vi "Build Message Configuration.vi"(8 "error in (no error)":errorcluster, 11 "Message XML Node":refnum<k20>) -> (0 "error out":errorcluster, 2 "Message  Config":T7={"Time to Next Msg (4 us)"=100, "Command Config"={"Command Type"=enum."Transmit", "Terminal Address"=enum."0", "SubAddress"=enum."Mode Code", "Word Count\\Mode Code"=enum."1", "Command Data"=[]}, "Message Control"={"MC17 Time Sync"=FALSE, "Error Mask"=FALSE, "Service Request Mask"=FALSE, "Busy Mask"=FALSE, "SubSystem Flag Mask"=FALSE, "Terminal Flag Mask"=FALSE, "Reserved Mask"=FALSE, "Retry"=FALSE, "Bus A / !Bus B"=FALSE, "Self-Test Loopback"=FALSE, "Broadcast Mask"=FALSE, "EoM Interrupt"=FALSE, "Mode Code Format"=FALSE, "Broadcast Format"=FALSE, "RT-RT Format"=FALSE}}, 3 "RT-RT Message Config":T1, 4 "RT-RT?":bool, 6 "Async?":bool)   [LabVIEW 2020]
doc: "Builds the various different flavors of Messages that can be defined by the XML. All Message types are handled here, including Asynchronous messages."
uses:
  Frames & Messages/TypeDefs/Message Config.ctl
  Frames & Messages/TypeDefs/Command Config.ctl
  Frames & Messages/TypeDefs/Command Type.ctl
  Frames & Messages/TypeDefs/Command Terminal Address.ctl
  Frames & Messages/TypeDefs/Command SubAddress.ctl
  Frames & Messages/TypeDefs/Command Word Count.ctl
  Frames & Messages/TypeDefs/Message Control.ctl
  Frames & Messages/TypeDefs/RT-RT Message Config.ctl
  BCI-1553 API.lvlib
  <vilib>/xml/NI_XML.lvlib
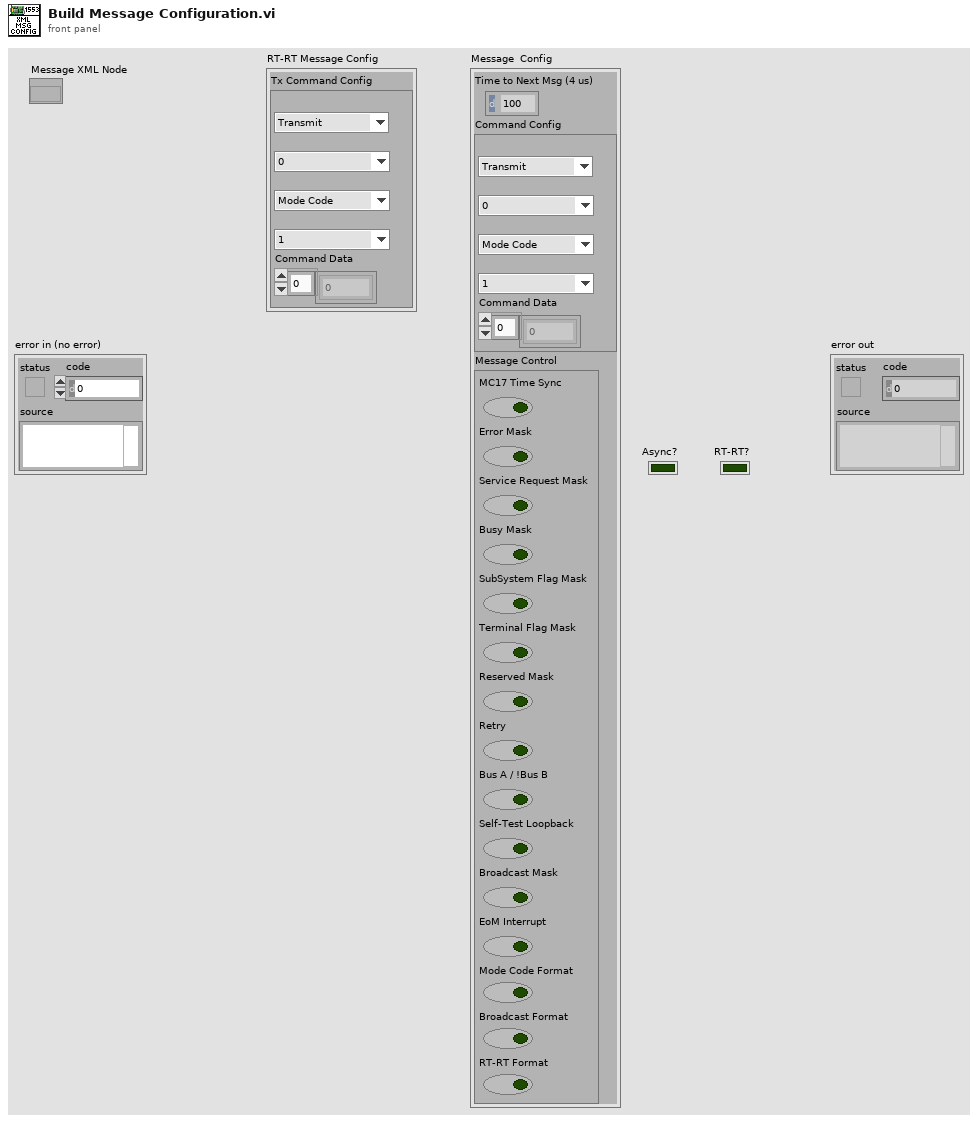
[diagram p1: front panel]
types:
  T1 = typedef "BCI-1553 API.lvlib/RT-RT Message Config.ctl" = cluster{"Tx Command Config":T2}
  T2 = typedef "BCI-1553 API.lvlib/Command Config.ctl" = cluster{"Command Type":T3, "Terminal Address":T4, "SubAddress":T5, "Word Count\\Mode Code":T6, "Command Data":u16[]}
  T3 = typedef "BCI-1553 API.lvlib/Command Type.ctl" = enum16{"Transmit", "Receive"}
  T4 = typedef "BCI-1553 API.lvlib/Command Terminal Address.ctl" = enum16{"0", "1", "2", "3", "4", "5", "6", "7", "8", "9", "10", "11", "12", "13", "14", "15", "16", "17", "18", "19", "20", "21", "22", "23", "24", "25", "26", "27", "28", "29", "30", "Broadcast"}
  T5 = typedef "BCI-1553 API.lvlib/Command SubAddress.ctl" = enum16{"Mode Code", "1", "2", "3", "4", "5", "6", "7", "8", "9", "10", "11", "12", "13", "14", "15", "16", "17", "18", "19", "20", "21", "22", "23", "24", "25", "26", "27", "28", "29", "30"}
  T6 = typedef "BCI-1553 API.lvlib/Command Word Count.ctl" = enum16{"1", "2", "3", "4", "5", "6", "7", "8", "9", "10", "11", "12", "13", "14", "15", "16", "17", "18", "19", "20", "21", "22", "23", "24", "25", "26", "27", "28", "29", "30", "31", "32"}
  T7 = typedef "BCI-1553 API.lvlib/Message Config.ctl" = cluster{"Time to Next Msg (4 us)":u16, "Command Config":T2, "Message Control":T8}
  T8 = typedef "BCI-1553 API.lvlib/Message Control.ctl" = cluster{"MC17 Time Sync":bool, "Error Mask":bool, "Service Request Mask":bool, "Busy Mask":bool, "SubSystem Flag Mask":bool, "Terminal Flag Mask":bool, "Reserved Mask":bool, "Retry":bool, "Bus A / !Bus B":bool, "Self-Test Loopback":bool, "Broadcast Mask":bool, "EoM Interrupt":bool, "Mode Code Format":bool, "Broadcast Format":bool, "RT-RT Format":bool}
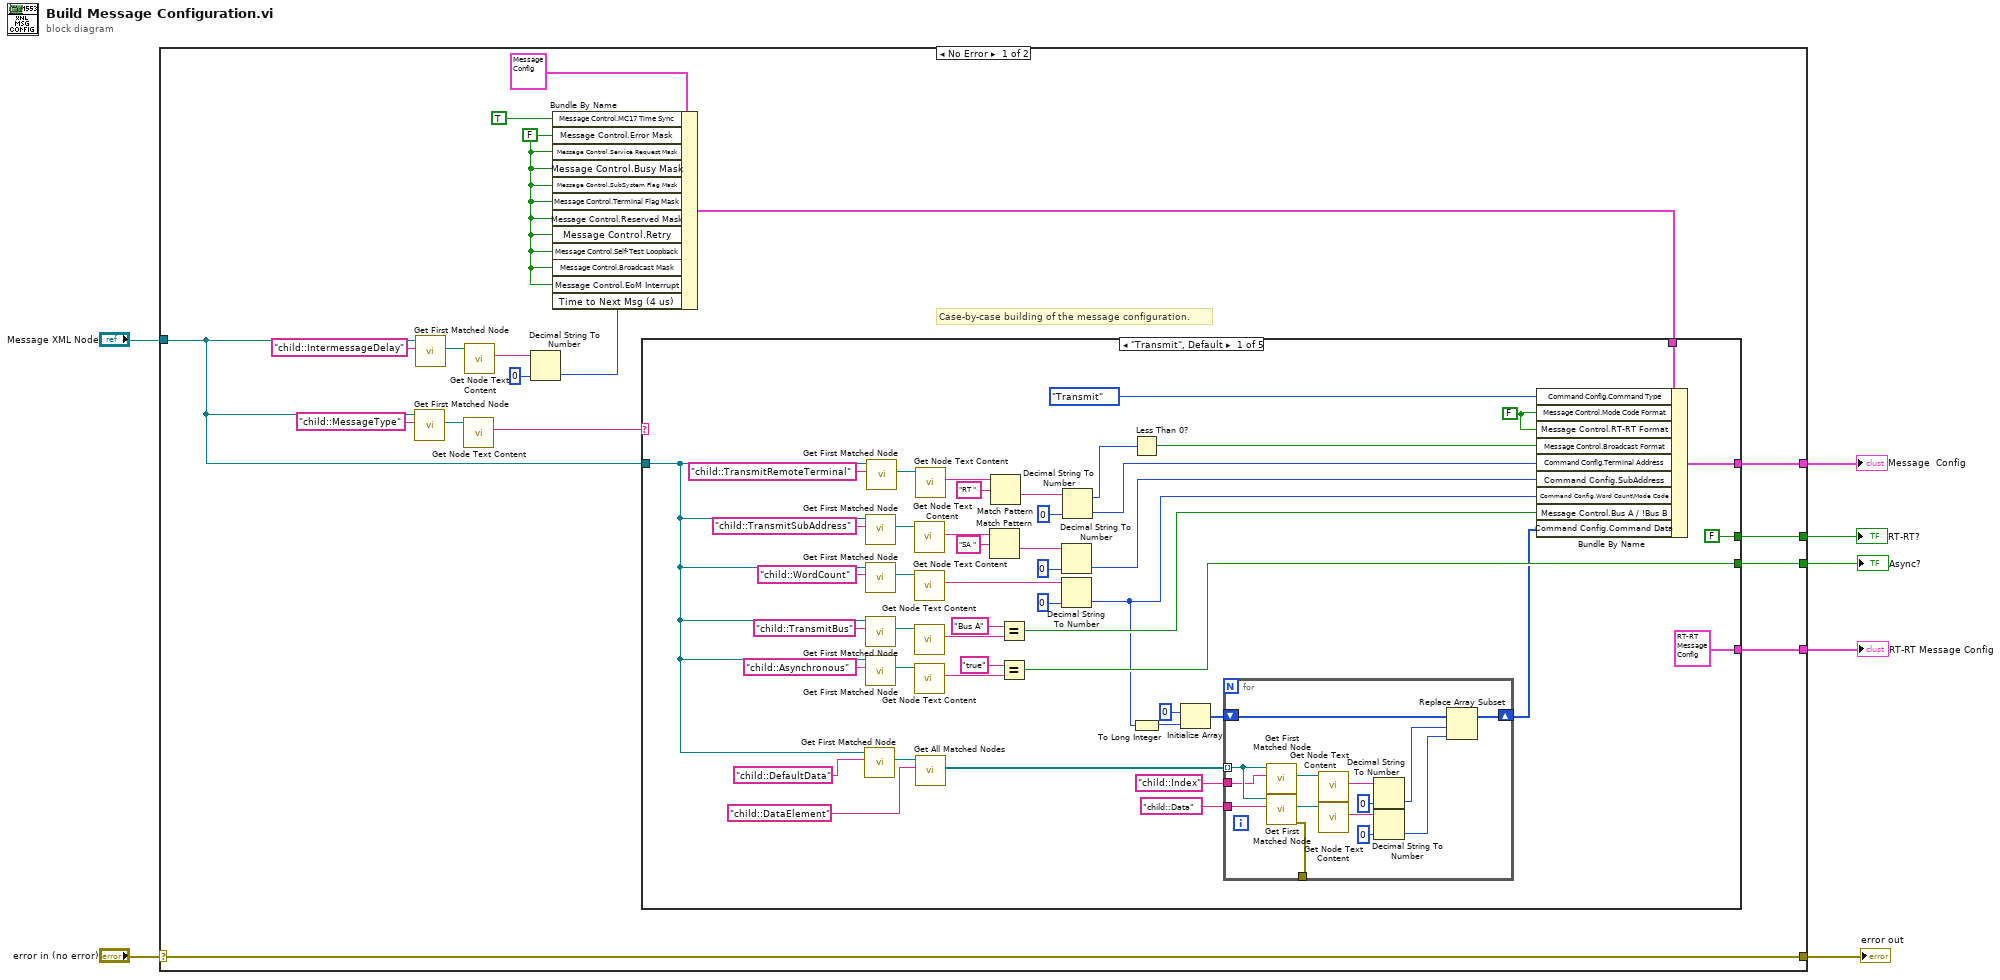
[diagram p0: block diagram]
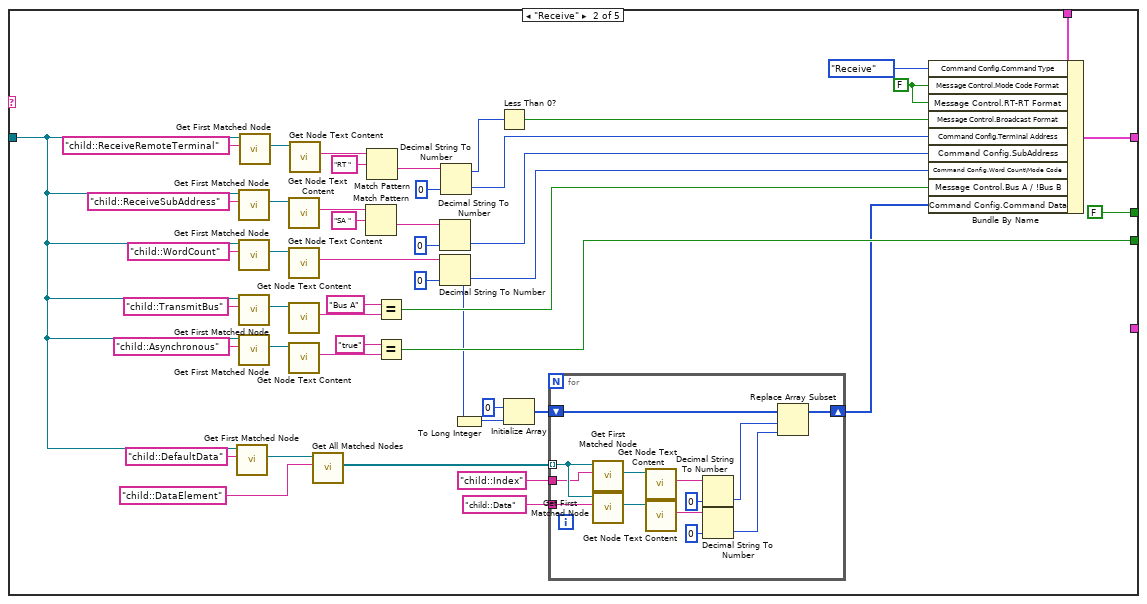
[diagram p2: hidden frame]
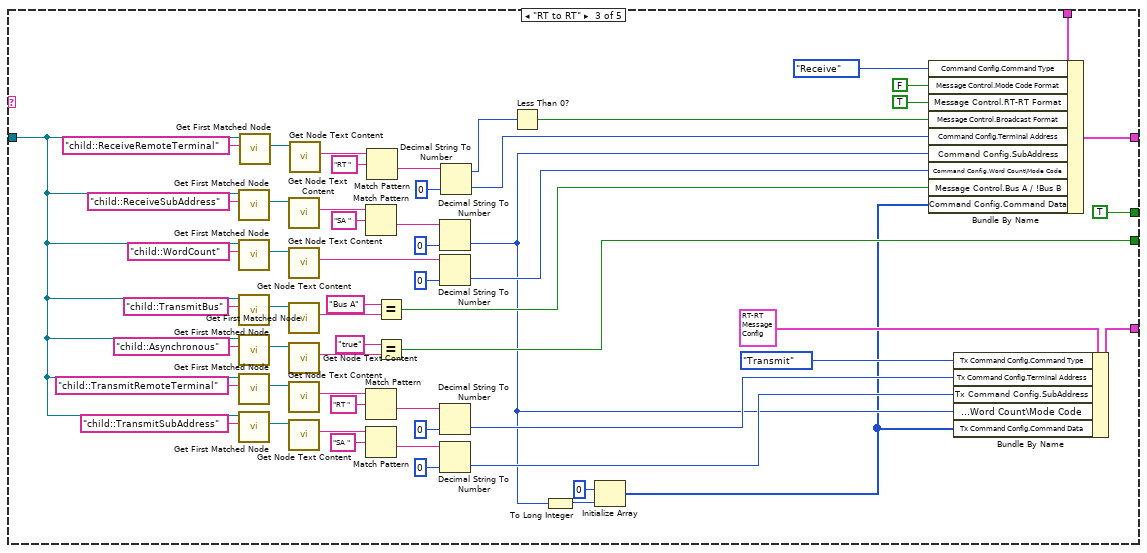
[diagram p3: hidden frame]
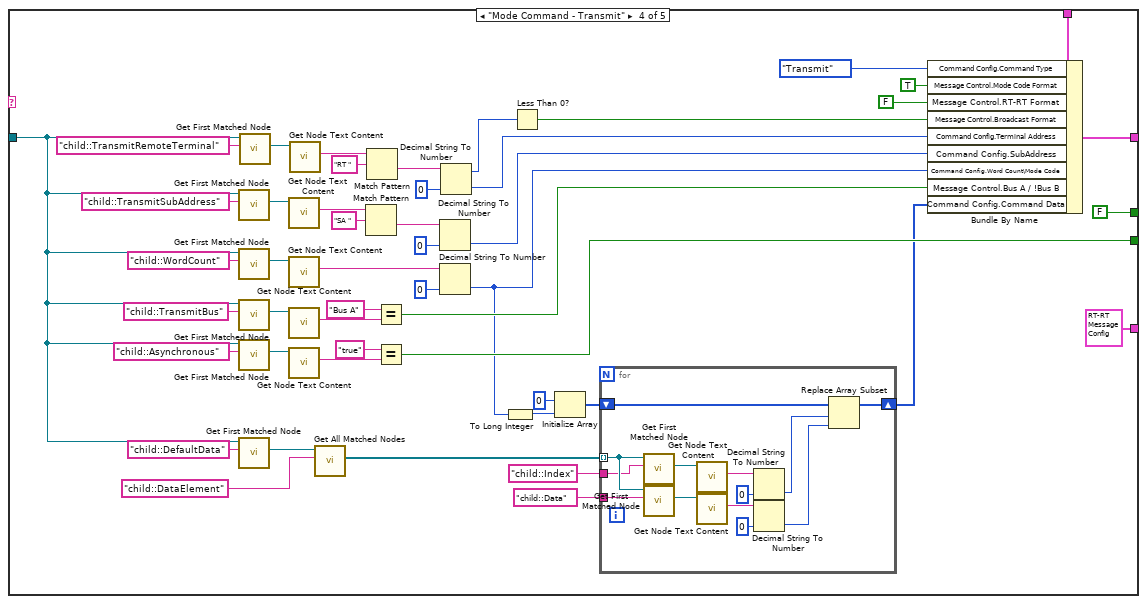
[diagram p4: hidden frame]
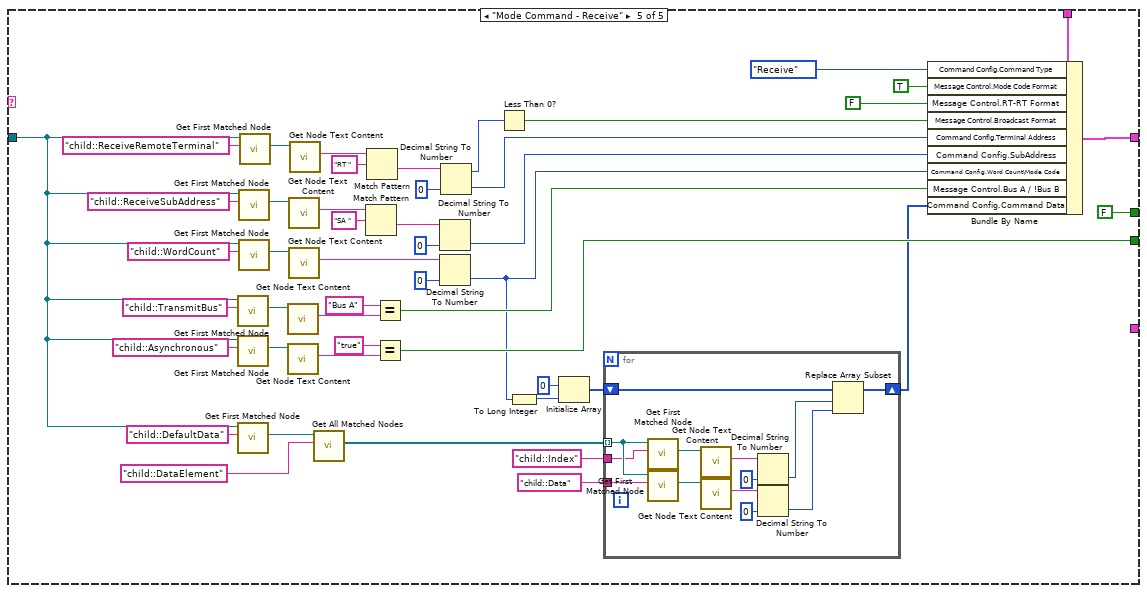
[diagram p5: hidden frame]
diagram:
  n1 = case shown="No Error" "error in (no error)" {
    selector: "error in (no error)" -> [w25 w329]
    tunnel: [w25 w329] -> w6
    tunnel: "Message XML Node" -> [w17 _]
    tunnel: [w14 _] -> w4
    tunnel: [w13 _] -> w3
    tunnel: [w12 _] -> w2
    tunnel: [w11 _] -> w1
    frame No Error {
      w8 = FALSE ("Message Control.Error Mask")
      # "Case-by-case building of the message configuration."
      n2 = call <vilib>:"Get First Matched Node.vi"("XPath expression"="child::MessageType", "node in"=w17) -> ("node result"=w19:refnum<k20>)  [unwired: 7 in, 2 out]
      n3 = call <vilib>:"Get First Matched Node.vi"("XPath expression"="child::IntermessageDelay", "node in"=w17) -> ("node result"=w22:refnum<k20>)  [unwired: 7 in, 2 out]
      n4 = call <vilib>:"Get Node Text Content.vi"("node in"=w19) -> ("node text"=w15:string)  [unwired: 8 in, 2 out]
      n5 = call <vilib>:"Get Node Text Content.vi"("node in"=w22) -> ("node text"=w21:string)  [unwired: 8 in, 2 out]
      n6 = Decimal String To Number(string=w21, default (0L)=u16 0 ("Time to Next Msg (100 us)")) -> (number=w10:u16)  [unwired: 1 in, 1 out]
      n7 = Bundle By Name(cluster=T7 {"Time to Next Msg (4 us)"=100, "Command Config"={"Command Type"=enum."Transmit", "Terminal Address"=enum."0", "SubAddress"=enum."Mode Code", "Word Count\\Mode Code"=enum."1", "Command Data"=[]}, "Message Control"={"MC17 Time Sync"=FALSE, "Error Mask"=FALSE, "Service Request Mask"=FALSE, "Busy Mask"=FALSE, "SubSystem Flag Mask"=FALSE, "Terminal Flag Mask"=FALSE, "Reserved Mask"=FALSE, "Retry"=FALSE, "Bus A / !Bus B"=FALSE, "Self-Test Loopback"=FALSE, "Broadcast Mask"=FALSE, "EoM Interrupt"=FALSE, "Mode Code Format"=FALSE, "Broadcast Format"=FALSE, "RT-RT Format"=FALSE}} ("Message  Config"), "Message Control.MC17 Time Sync"=TRUE, "Message Control.Error Mask"=w8, "Message Control.Service Request Mask"=w8, "Message Control.Busy Mask"=w8, "Message Control.SubSystem Flag Mask"=w8, "Message Control.Terminal Flag Mask"=w8, "Message Control.Reserved Mask"=w8, "Message Control.Retry"=w8, "Message Control.Self-Test Loopback"=w8, "Message Control.Broadcast Mask"=w8, "Message Control.EoM Interrupt"=w8, "Time to Next Msg (4 us)"=w10) -> (w16:T7)
      n8 = case shown="\"Transmit\", Default" w15 {
        tunnel: w17 -> [w26 w98 w156 w206 w270]
        tunnel: w16 -> [w60 w122 w192 w241 w303]
        tunnel: [FALSE FALSE TRUE FALSE FALSE] -> w14
        tunnel: [w55 w116 w188 w236 w297] -> w13
        tunnel: [T1 {"Tx Command Config"={"Command Type"=enum."Transmit", "Terminal Address"=enum."0", "SubAddress"=enum."Mode Code", "Word Count\\Mode Code"=enum."1", "Command Data"=[]}} ("RT-RT Message Config") _ w168 T1 {"Tx Command Config"={"Command Type"=enum."Transmit", "Terminal Address"=enum."0", "SubAddress"=enum."Mode Code", "Word Count\\Mode Code"=enum."1", "Command Data"=[]}} ("RT-RT Message Config") _] -> w12
        tunnel: [w38 w100 w171 w219 w281] -> w11
        frame "Transmit", Default {
          w59 = FALSE ("Message Control.Mode Code Format")
          n9 = call <vilib>:"Get First Matched Node.vi"("XPath expression"="child::DefaultData", "node in"=w26) -> ("node result"=w30:refnum<k20>)  [unwired: 7 in, 2 out]
          n10 = call <vilib>:"Get First Matched Node.vi"("XPath expression"="child::TransmitSubAddress", "node in"=w26) -> ("node result"=w63:refnum<k20>)  [unwired: 7 in, 2 out]
          n11 = call <vilib>:"Get First Matched Node.vi"("XPath expression"="child::WordCount", "node in"=w26) -> ("node result"=w50:refnum<k20>)  [unwired: 7 in, 2 out]
          n12 = call <vilib>:"Get First Matched Node.vi"("XPath expression"="child::TransmitBus", "node in"=w26) -> ("node result"=w44:refnum<k20>)  [unwired: 7 in, 2 out]
          n13 = call <vilib>:"Get First Matched Node.vi"("XPath expression"="child::Asynchronous", "node in"=w26) -> ("node result"=w47:refnum<k20>)  [unwired: 7 in, 2 out]
          n14 = call <vilib>:"Get First Matched Node.vi"("XPath expression"="child::TransmitRemoteTerminal", "node in"=w26) -> ("node result"=w72:refnum<k20>)  [unwired: 7 in, 2 out]
          n15 = call <vilib>:"Get Node Text Content.vi"("node in"=w63) -> ("node text"=w64:string)  [unwired: 8 in, 2 out]
          n16 = call <vilib>:"Get Node Text Content.vi"("node in"=w50) -> ("node text"=w48:string)  [unwired: 8 in, 2 out]
          n17 = call <vilib>:"Get Node Text Content.vi"("node in"=w44) -> ("node text"=w43:string)  [unwired: 8 in, 2 out]
          n18 = call <vilib>:"Get Node Text Content.vi"("node in"=w47) -> ("node text"=w41:string)  [unwired: 8 in, 2 out]
          n19 = call <vilib>:"Get Node Text Content.vi"("node in"=w72) -> ("node text"=w71:string)  [unwired: 8 in, 2 out]
          n20 = call <vilib>:"Get All Matched Nodes.vi"("XPath expression"="child::DataElement", "node in"=w30) -> ("node result array"=w37:refnum<k20>[])  [unwired: 7 in, 2 out]
          n21 = Match Pattern(string=w64, regular expression="SA " ("x")) -> (after substring=w66:string)  [unwired: 1 in, 3 out]
          n22 = Match Pattern(string=w71, regular expression="RT " ("x")) -> (after substring=w69:string)  [unwired: 1 in, 3 out]
          n23 = Equal?(x="Bus A", y=w43) -> (x = y?=w39:bool)
          n24 = Equal?(x="true", y=w41) -> (x = y?=w38:bool)
          n25 = Decimal String To Number(string=w66, default (0L)=u16 0 ("Command Config.Terminal Address (0-30)")) -> (number=w57:u16)  [unwired: 1 in, 1 out]
          n26 = Decimal String To Number(string=w48, default (0L)=u16 0 ("Command Config.Terminal Address (0-30)")) -> (number=w27:u16)  [unwired: 1 in, 1 out]
          n27 = Decimal String To Number(string=w69, default (0L)=u16 0 ("Command Config.Terminal Address (0-30)")) -> (offset past number=w52:i32, number=w58:u16)  [unwired: 1 in]
          n28 = Less Than 0?(x=w52) -> (x < 0?=w53:bool)
          n29 = To Long Integer(number=w27) -> (32bit integer=w33:i32)
          n30 = Initialize Array(u16 0 ("element"), w33) -> (w32:u16[])
          n31 = for {
            tunnel: w37 -> [w85] mode=indexing
            shift-right: [w86] -> w28
            shift-left: w32 -> [w87]
            tunnel: "child::Index" ("XPath expression") -> [w84]
            tunnel: "child::Data" ("XPath expression") -> [w83]
            tunnel: [w74] -> _
            n32 = call <vilib>:"Get First Matched Node.vi"("XPath expression"=w84, "node in"=w85) -> ("node result"=w82:refnum<k20>)  [unwired: 7 in, 2 out]
            n33 = call <vilib>:"Get First Matched Node.vi"("XPath expression"=w83, "node in"=w85) -> ("error out"=w74:errorcluster, "node result"=w81:refnum<k20>)  [unwired: 7 in, 1 out]
            n34 = call <vilib>:"Get Node Text Content.vi"("node in"=w82) -> ("node text"=w78:string)  [unwired: 8 in, 2 out]
            n35 = call <vilib>:"Get Node Text Content.vi"("node in"=w81) -> ("node text"=w77:string)  [unwired: 8 in, 2 out]
            n36 = Decimal String To Number(string=w78, default (0L)=0 ("Command Config.Terminal Address (0-30)")) -> (number=w76:i32)  [unwired: 1 in, 1 out]
            n37 = Decimal String To Number(string=w77, default (0L)=u16 0 ("Command Config.Terminal Address (0-30)")) -> (number=w75:u16)  [unwired: 1 in, 1 out]
            n38 = Replace Array Subset(array=w87, new element=w75, index=w76) -> (w86:u16[])
          }
          n39 = Bundle By Name(cluster=w60, "Command Config.Command Type"=enum16{"Transmit", "Receive"}."Transmit", "Message Control.Mode Code Format"=w59, "Message Control.RT-RT Format"=w59, "Message Control.Broadcast Format"=w53, "Command Config.Terminal Address"=w58, "Command Config.SubAddress"=w57, "Command Config.Word Count\\Mode Code"=w27, "Message Control.Bus A / !Bus B"=w39, "Command Config.Command Data"=w28) -> (w55:T7)
        }
        frame "Receive" {
          w120 = FALSE ("Message Control.Mode Code Format")
          n40 = call <vilib>:"Get First Matched Node.vi"("XPath expression"="child::DefaultData", "node in"=w98) -> ("node result"=w97:refnum<k20>)  [unwired: 7 in, 2 out]
          n41 = call <vilib>:"Get First Matched Node.vi"("XPath expression"="child::ReceiveSubAddress", "node in"=w98) -> ("node result"=w124:refnum<k20>)  [unwired: 7 in, 2 out]
          n42 = call <vilib>:"Get First Matched Node.vi"("XPath expression"="child::WordCount", "node in"=w98) -> ("node result"=w112:refnum<k20>)  [unwired: 7 in, 2 out]
          n43 = call <vilib>:"Get First Matched Node.vi"("XPath expression"="child::TransmitBus", "node in"=w98) -> ("node result"=w106:refnum<k20>)  [unwired: 7 in, 2 out]
          n44 = call <vilib>:"Get First Matched Node.vi"("XPath expression"="child::Asynchronous", "node in"=w98) -> ("node result"=w109:refnum<k20>)  [unwired: 7 in, 2 out]
          n45 = call <vilib>:"Get First Matched Node.vi"("XPath expression"="child::ReceiveRemoteTerminal", "node in"=w98) -> ("node result"=w133:refnum<k20>)  [unwired: 7 in, 2 out]
          n46 = call <vilib>:"Get Node Text Content.vi"("node in"=w124) -> ("node text"=w125:string)  [unwired: 8 in, 2 out]
          n47 = call <vilib>:"Get Node Text Content.vi"("node in"=w112) -> ("node text"=w110:string)  [unwired: 8 in, 2 out]
          n48 = call <vilib>:"Get Node Text Content.vi"("node in"=w106) -> ("node text"=w105:string)  [unwired: 8 in, 2 out]
          n49 = call <vilib>:"Get Node Text Content.vi"("node in"=w109) -> ("node text"=w102:string)  [unwired: 8 in, 2 out]
          n50 = call <vilib>:"Get Node Text Content.vi"("node in"=w133) -> ("node text"=w132:string)  [unwired: 8 in, 2 out]
          n51 = call <vilib>:"Get All Matched Nodes.vi"("XPath expression"="child::DataElement", "node in"=w97) -> ("node result array"=w95:refnum<k20>[])  [unwired: 7 in, 2 out]
          n52 = Match Pattern(string=w125, regular expression="SA " ("x")) -> (after substring=w127:string)  [unwired: 1 in, 3 out]
          n53 = Match Pattern(string=w132, regular expression="RT " ("x")) -> (after substring=w130:string)  [unwired: 1 in, 3 out]
          n54 = Equal?(x="Bus A", y=w105) -> (x = y?=w103:bool)
          n55 = Equal?(x="true", y=w102) -> (x = y?=w100:bool)
          n56 = Decimal String To Number(string=w127, default (0L)=u16 0 ("Command Config.Terminal Address (0-30)")) -> (number=w118:u16)  [unwired: 1 in, 1 out]
          n57 = Decimal String To Number(string=w110, default (0L)=u16 0 ("Command Config.Terminal Address (0-30)")) -> (number=w94:u16)  [unwired: 1 in, 1 out]
          n58 = Decimal String To Number(string=w130, default (0L)=u16 0 ("Command Config.Terminal Address (0-30)")) -> (offset past number=w114:i32, number=w119:u16)  [unwired: 1 in]
          n59 = To Long Integer(number=w94) -> (32bit integer=w92:i32)
          n60 = Less Than 0?(x=w114) -> (x < 0?=w115:bool)
          n61 = Initialize Array(u16 0 ("element"), w92) -> (w93:u16[])
          n62 = for {
            tunnel: w95 -> [w145] mode=indexing
            shift-right: [w146] -> w90
            shift-left: w93 -> [w147]
            tunnel: "child::Index" ("XPath expression") -> [w144]
            tunnel: "child::Data" ("XPath expression") -> [w143]
            n63 = call <vilib>:"Get First Matched Node.vi"("XPath expression"=w144, "node in"=w145) -> ("node result"=w142:refnum<k20>)  [unwired: 7 in, 2 out]
            n64 = call <vilib>:"Get First Matched Node.vi"("XPath expression"=w143, "node in"=w145) -> ("node result"=w141:refnum<k20>)  [unwired: 7 in, 2 out]
            n65 = call <vilib>:"Get Node Text Content.vi"("node in"=w142) -> ("node text"=w138:string)  [unwired: 8 in, 2 out]
            n66 = call <vilib>:"Get Node Text Content.vi"("node in"=w141) -> ("node text"=w137:string)  [unwired: 8 in, 2 out]
            n67 = Decimal String To Number(string=w138, default (0L)=0 ("Command Config.Terminal Address (0-30)")) -> (number=w136:i32)  [unwired: 1 in, 1 out]
            n68 = Decimal String To Number(string=w137, default (0L)=u16 0 ("Command Config.Terminal Address (0-30)")) -> (number=w135:u16)  [unwired: 1 in, 1 out]
            n69 = Replace Array Subset(array=w147, new element=w135, index=w136) -> (w146:u16[])
          }
          n70 = Bundle By Name(cluster=w122, "Command Config.Command Type"=enum16{"Transmit", "Receive"}."Receive", "Message Control.Mode Code Format"=w120, "Message Control.RT-RT Format"=w120, "Message Control.Broadcast Format"=w115, "Command Config.Terminal Address"=w119, "Command Config.SubAddress"=w118, "Command Config.Word Count\\Mode Code"=w94, "Message Control.Bus A / !Bus B"=w103, "Command Config.Command Data"=w90) -> (w116:T7)
        }
        frame "RT to RT" {
          n71 = call <vilib>:"Get First Matched Node.vi"("XPath expression"="child::ReceiveSubAddress", "node in"=w156) -> ("node result"=w195:refnum<k20>)  [unwired: 7 in, 2 out]
          n72 = call <vilib>:"Get First Matched Node.vi"("XPath expression"="child::WordCount", "node in"=w156) -> ("node result"=w184:refnum<k20>)  [unwired: 7 in, 2 out]
          n73 = call <vilib>:"Get First Matched Node.vi"("XPath expression"="child::TransmitBus", "node in"=w156) -> ("node result"=w177:refnum<k20>)  [unwired: 7 in, 2 out]
          n74 = call <vilib>:"Get First Matched Node.vi"("XPath expression"="child::Asynchronous", "node in"=w156) -> ("node result"=w180:refnum<k20>)  [unwired: 7 in, 2 out]
          n75 = call <vilib>:"Get First Matched Node.vi"("XPath expression"="child::TransmitRemoteTerminal", "node in"=w156) -> ("node result"=w158:refnum<k20>)  [unwired: 7 in, 2 out]
          n76 = call <vilib>:"Get First Matched Node.vi"("XPath expression"="child::TransmitSubAddress", "node in"=w156) -> ("node result"=w166:refnum<k20>)  [unwired: 7 in, 2 out]
          n77 = call <vilib>:"Get First Matched Node.vi"("XPath expression"="child::ReceiveRemoteTerminal", "node in"=w156) -> ("node result"=w204:refnum<k20>)  [unwired: 7 in, 2 out]
          n78 = call <vilib>:"Get Node Text Content.vi"("node in"=w195) -> ("node text"=w196:string)  [unwired: 8 in, 2 out]
          n79 = call <vilib>:"Get Node Text Content.vi"("node in"=w184) -> ("node text"=w182:string)  [unwired: 8 in, 2 out]
          n80 = call <vilib>:"Get Node Text Content.vi"("node in"=w177) -> ("node text"=w176:string)  [unwired: 8 in, 2 out]
          n81 = call <vilib>:"Get Node Text Content.vi"("node in"=w180) -> ("node text"=w174:string)  [unwired: 8 in, 2 out]
          n82 = call <vilib>:"Get Node Text Content.vi"("node in"=w158) -> ("node text"=w159:string)  [unwired: 8 in, 2 out]
          n83 = call <vilib>:"Get Node Text Content.vi"("node in"=w166) -> ("node text"=w165:string)  [unwired: 8 in, 2 out]
          n84 = call <vilib>:"Get Node Text Content.vi"("node in"=w204) -> ("node text"=w203:string)  [unwired: 8 in, 2 out]
          n85 = Match Pattern(string=w196, regular expression="SA " ("x")) -> (after substring=w198:string)  [unwired: 1 in, 3 out]
          n86 = Match Pattern(string=w159, regular expression="RT " ("x")) -> (after substring=w161:string)  [unwired: 1 in, 3 out]
          n87 = Match Pattern(string=w165, regular expression="SA " ("x")) -> (after substring=w163:string)  [unwired: 1 in, 3 out]
          n88 = Match Pattern(string=w203, regular expression="RT " ("x")) -> (after substring=w201:string)  [unwired: 1 in, 3 out]
          n89 = Equal?(x="Bus A", y=w176) -> (x = y?=w172:bool)
          n90 = Equal?(x="true", y=w174) -> (x = y?=w171:bool)
          n91 = Decimal String To Number(string=w198, default (0L)=u16 0 ("Command Config.Terminal Address (0-30)")) -> (number=w149:u16)  [unwired: 1 in, 1 out]
          n92 = Decimal String To Number(string=w182, default (0L)=u16 0 ("Command Config.Terminal Address (0-30)")) -> (number=w181:u16)  [unwired: 1 in, 1 out]
          n93 = Decimal String To Number(string=w161, default (0L)=u16 0 ("Command Config.Terminal Address (0-30)")) -> (number=w153:u16)  [unwired: 1 in, 1 out]
          n94 = Decimal String To Number(string=w163, default (0L)=u16 0 ("Command Config.Terminal Address (0-30)")) -> (number=w154:u16)  [unwired: 1 in, 1 out]
          n95 = Decimal String To Number(string=w201, default (0L)=u16 0 ("Command Config.Terminal Address (0-30)")) -> (offset past number=w186:i32, number=w190:u16)  [unwired: 1 in]
          n96 = Less Than 0?(x=w186) -> (x < 0?=w187:bool)
          n97 = To Long Integer(number=w149) -> (32bit integer=w150:i32)
          n98 = Initialize Array(u16 0 ("element"), w150) -> (w148:u16[])
          n99 = Bundle By Name(cluster=w192, "Command Config.Command Type"=enum16{"Transmit", "Receive"}."Receive", "Message Control.Mode Code Format"=FALSE, "Message Control.RT-RT Format"=TRUE, "Message Control.Broadcast Format"=w187, "Command Config.Terminal Address"=w190, "Command Config.SubAddress"=w149, "Command Config.Word Count\\Mode Code"=w181, "Message Control.Bus A / !Bus B"=w172, "Command Config.Command Data"=w148) -> (w188:T7)
          n100 = Bundle By Name(cluster=T1 {"Tx Command Config"={"Command Type"=enum."Transmit", "Terminal Address"=enum."0", "SubAddress"=enum."Mode Code", "Word Count\\Mode Code"=enum."1", "Command Data"=[]}} ("RT-RT Message Config"), "Tx Command Config.Command Type"=enum16{"Transmit", "Receive"}."Transmit", "Tx Command Config.Terminal Address"=w153, "Tx Command Config.SubAddress"=w154, "Tx Command Config.Word Count\\Mode Code"=w149, "Tx Command Config.Command Data"=w148) -> (w168:T1)
        }
        frame "Mode Command - Transmit" {
          n101 = call <vilib>:"Get First Matched Node.vi"("XPath expression"="child::TransmitSubAddress", "node in"=w206) -> ("node result"=w244:refnum<k20>)  [unwired: 7 in, 2 out]
          n102 = call <vilib>:"Get First Matched Node.vi"("XPath expression"="child::WordCount", "node in"=w206) -> ("node result"=w231:refnum<k20>)  [unwired: 7 in, 2 out]
          n103 = call <vilib>:"Get First Matched Node.vi"("XPath expression"="child::TransmitBus", "node in"=w206) -> ("node result"=w225:refnum<k20>)  [unwired: 7 in, 2 out]
          n104 = call <vilib>:"Get First Matched Node.vi"("XPath expression"="child::Asynchronous", "node in"=w206) -> ("node result"=w228:refnum<k20>)  [unwired: 7 in, 2 out]
          n105 = call <vilib>:"Get First Matched Node.vi"("XPath expression"="child::DefaultData", "node in"=w206) -> ("node result"=w210:refnum<k20>)  [unwired: 7 in, 2 out]
          n106 = call <vilib>:"Get First Matched Node.vi"("XPath expression"="child::TransmitRemoteTerminal", "node in"=w206) -> ("node result"=w253:refnum<k20>)  [unwired: 7 in, 2 out]
          n107 = call <vilib>:"Get Node Text Content.vi"("node in"=w244) -> ("node text"=w245:string)  [unwired: 8 in, 2 out]
          n108 = call <vilib>:"Get Node Text Content.vi"("node in"=w231) -> ("node text"=w229:string)  [unwired: 8 in, 2 out]
          n109 = call <vilib>:"Get Node Text Content.vi"("node in"=w225) -> ("node text"=w224:string)  [unwired: 8 in, 2 out]
          n110 = call <vilib>:"Get Node Text Content.vi"("node in"=w228) -> ("node text"=w222:string)  [unwired: 8 in, 2 out]
          n111 = call <vilib>:"Get Node Text Content.vi"("node in"=w253) -> ("node text"=w252:string)  [unwired: 8 in, 2 out]
          n112 = call <vilib>:"Get All Matched Nodes.vi"("XPath expression"="child::DataElement", "node in"=w210) -> ("node result array"=w217:refnum<k20>[])  [unwired: 7 in, 2 out]
          n113 = Match Pattern(string=w245, regular expression="SA " ("x")) -> (after substring=w247:string)  [unwired: 1 in, 3 out]
          n114 = Match Pattern(string=w252, regular expression="RT " ("x")) -> (after substring=w250:string)  [unwired: 1 in, 3 out]
          n115 = Equal?(x="Bus A", y=w224) -> (x = y?=w220:bool)
          n116 = Equal?(x="true", y=w222) -> (x = y?=w219:bool)
          n117 = Decimal String To Number(string=w247, default (0L)=u16 0 ("Command Config.Terminal Address (0-30)")) -> (number=w238:u16)  [unwired: 1 in, 1 out]
          n118 = Decimal String To Number(string=w229, default (0L)=u16 0 ("Command Config.Terminal Address (0-30)")) -> (number=w207:u16)  [unwired: 1 in, 1 out]
          n119 = Decimal String To Number(string=w250, default (0L)=u16 0 ("Command Config.Terminal Address (0-30)")) -> (offset past number=w233:i32, number=w239:u16)  [unwired: 1 in]
          n120 = To Long Integer(number=w207) -> (32bit integer=w213:i32)
          n121 = Less Than 0?(x=w233) -> (x < 0?=w234:bool)
          n122 = Initialize Array(u16 0 ("element"), w213) -> (w212:u16[])
          n123 = for {
            tunnel: w217 -> [w265] mode=indexing
            shift-right: [w266] -> w208
            shift-left: w212 -> [w267]
            tunnel: "child::Index" ("XPath expression") -> [w264]
            tunnel: "child::Data" ("XPath expression") -> [w263]
            n124 = call <vilib>:"Get First Matched Node.vi"("XPath expression"=w264, "node in"=w265) -> ("node result"=w262:refnum<k20>)  [unwired: 7 in, 2 out]
            n125 = call <vilib>:"Get First Matched Node.vi"("XPath expression"=w263, "node in"=w265) -> ("node result"=w261:refnum<k20>)  [unwired: 7 in, 2 out]
            n126 = call <vilib>:"Get Node Text Content.vi"("node in"=w262) -> ("node text"=w258:string)  [unwired: 8 in, 2 out]
            n127 = call <vilib>:"Get Node Text Content.vi"("node in"=w261) -> ("node text"=w257:string)  [unwired: 8 in, 2 out]
            n128 = Decimal String To Number(string=w258, default (0L)=0 ("Command Config.Terminal Address (0-30)")) -> (number=w256:i32)  [unwired: 1 in, 1 out]
            n129 = Decimal String To Number(string=w257, default (0L)=u16 0 ("Command Config.Terminal Address (0-30)")) -> (number=w255:u16)  [unwired: 1 in, 1 out]
            n130 = Replace Array Subset(array=w267, new element=w255, index=w256) -> (w266:u16[])
          }
          n131 = Bundle By Name(cluster=w241, "Command Config.Command Type"=enum16{"Transmit", "Receive"}."Transmit", "Message Control.Mode Code Format"=TRUE, "Message Control.RT-RT Format"=FALSE ("Message Control.Mode Code Format"), "Message Control.Broadcast Format"=w234, "Command Config.Terminal Address"=w239, "Command Config.SubAddress"=w238, "Command Config.Word Count\\Mode Code"=w207, "Message Control.Bus A / !Bus B"=w220, "Command Config.Command Data"=w208) -> (w236:T7)
        }
        frame "Mode Command - Receive" {
          n132 = call <vilib>:"Get First Matched Node.vi"("XPath expression"="child::TransmitBus", "node in"=w270) -> ("node result"=w287:refnum<k20>)  [unwired: 7 in, 2 out]
          n133 = call <vilib>:"Get First Matched Node.vi"("XPath expression"="child::Asynchronous", "node in"=w270) -> ("node result"=w290:refnum<k20>)  [unwired: 7 in, 2 out]
          n134 = call <vilib>:"Get First Matched Node.vi"("XPath expression"="child::DefaultData", "node in"=w270) -> ("node result"=w272:refnum<k20>)  [unwired: 7 in, 2 out]
          n135 = call <vilib>:"Get First Matched Node.vi"("XPath expression"="child::ReceiveSubAddress", "node in"=w270) -> ("node result"=w305:refnum<k20>)  [unwired: 7 in, 2 out]
          n136 = call <vilib>:"Get First Matched Node.vi"("XPath expression"="child::WordCount", "node in"=w270) -> ("node result"=w293:refnum<k20>)  [unwired: 7 in, 2 out]
          n137 = call <vilib>:"Get First Matched Node.vi"("XPath expression"="child::ReceiveRemoteTerminal", "node in"=w270) -> ("node result"=w314:refnum<k20>)  [unwired: 7 in, 2 out]
          n138 = call <vilib>:"Get Node Text Content.vi"("node in"=w287) -> ("node text"=w286:string)  [unwired: 8 in, 2 out]
          n139 = call <vilib>:"Get Node Text Content.vi"("node in"=w290) -> ("node text"=w283:string)  [unwired: 8 in, 2 out]
          n140 = call <vilib>:"Get Node Text Content.vi"("node in"=w305) -> ("node text"=w306:string)  [unwired: 8 in, 2 out]
          n141 = call <vilib>:"Get Node Text Content.vi"("node in"=w293) -> ("node text"=w291:string)  [unwired: 8 in, 2 out]
          n142 = call <vilib>:"Get Node Text Content.vi"("node in"=w314) -> ("node text"=w313:string)  [unwired: 8 in, 2 out]
          n143 = call <vilib>:"Get All Matched Nodes.vi"("XPath expression"="child::DataElement", "node in"=w272) -> ("node result array"=w279:refnum<k20>[])  [unwired: 7 in, 2 out]
          n144 = Match Pattern(string=w306, regular expression="SA " ("x")) -> (after substring=w308:string)  [unwired: 1 in, 3 out]
          n145 = Match Pattern(string=w313, regular expression="RT " ("x")) -> (after substring=w311:string)  [unwired: 1 in, 3 out]
          n146 = Equal?(x="Bus A", y=w286) -> (x = y?=w284:bool)
          n147 = Equal?(x="true", y=w283) -> (x = y?=w281:bool)
          n148 = Decimal String To Number(string=w308, default (0L)=u16 0 ("Command Config.Terminal Address (0-30)")) -> (number=w299:u16)  [unwired: 1 in, 1 out]
          n149 = Decimal String To Number(string=w291, default (0L)=u16 0 ("Command Config.Terminal Address (0-30)")) -> (number=w269:u16)  [unwired: 1 in, 1 out]
          n150 = Decimal String To Number(string=w311, default (0L)=u16 0 ("Command Config.Terminal Address (0-30)")) -> (offset past number=w295:i32, number=w300:u16)  [unwired: 1 in]
          n151 = Less Than 0?(x=w295) -> (x < 0?=w296:bool)
          n152 = To Long Integer(number=w269) -> (32bit integer=w275:i32)
          n153 = Initialize Array(u16 0 ("element"), w275) -> (w274:u16[])
          n154 = for {
            tunnel: w279 -> [w326] mode=indexing
            shift-right: [w327] -> w268
            shift-left: w274 -> [w328]
            tunnel: "child::Index" ("XPath expression") -> [w325]
            tunnel: "child::Data" ("XPath expression") -> [w324]
            n155 = call <vilib>:"Get First Matched Node.vi"("XPath expression"=w325, "node in"=w326) -> ("node result"=w323:refnum<k20>)  [unwired: 7 in, 2 out]
            n156 = call <vilib>:"Get First Matched Node.vi"("XPath expression"=w324, "node in"=w326) -> ("node result"=w322:refnum<k20>)  [unwired: 7 in, 2 out]
            n157 = call <vilib>:"Get Node Text Content.vi"("node in"=w323) -> ("node text"=w319:string)  [unwired: 8 in, 2 out]
            n158 = call <vilib>:"Get Node Text Content.vi"("node in"=w322) -> ("node text"=w318:string)  [unwired: 8 in, 2 out]
            n159 = Decimal String To Number(string=w319, default (0L)=0 ("Command Config.Terminal Address (0-30)")) -> (number=w317:i32)  [unwired: 1 in, 1 out]
            n160 = Decimal String To Number(string=w318, default (0L)=u16 0 ("Command Config.Terminal Address (0-30)")) -> (number=w316:u16)  [unwired: 1 in, 1 out]
            n161 = Replace Array Subset(array=w328, new element=w316, index=w317) -> (w327:u16[])
          }
          n162 = Bundle By Name(cluster=w303, "Command Config.Command Type"=enum16{"Transmit", "Receive"}."Receive", "Message Control.Mode Code Format"=TRUE, "Message Control.RT-RT Format"=FALSE ("Message Control.Mode Code Format"), "Message Control.Broadcast Format"=w296, "Command Config.Terminal Address"=w300, "Command Config.SubAddress"=w299, "Command Config.Word Count\\Mode Code"=w269, "Message Control.Bus A / !Bus B"=w284, "Command Config.Command Data"=w268) -> (w297:T7)
        }
      }
    }
    frame Error {
    }
  }
  "error out" <- w6
  "Message  Config" <- w3
  "RT-RT?" <- w4
  "RT-RT Message Config" <- w2
  "Async?" <- w1
